vi "Get 12-bit image array.vi"(7 "Error In":errorcluster, 8 "Height":i32=2054, 9 "Width":i32=2456, 10 "Camera reference in":refnum<k24>) -> (0 "Error Out":errorcluster, 2 "Array":u16[][](array[numeric]), 3 "Camera reference out":refnum<k24>)   [LabVIEW 2017]
uses:
  C:/Program Files/National Instruments/LabVIEW 2017/instr.lib/IDS/ueye.NET/uEyeDotNet.dll
panel:
  out "Cam read time":u32
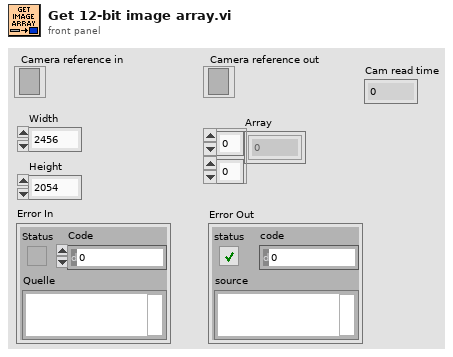
[diagram p1: front panel]
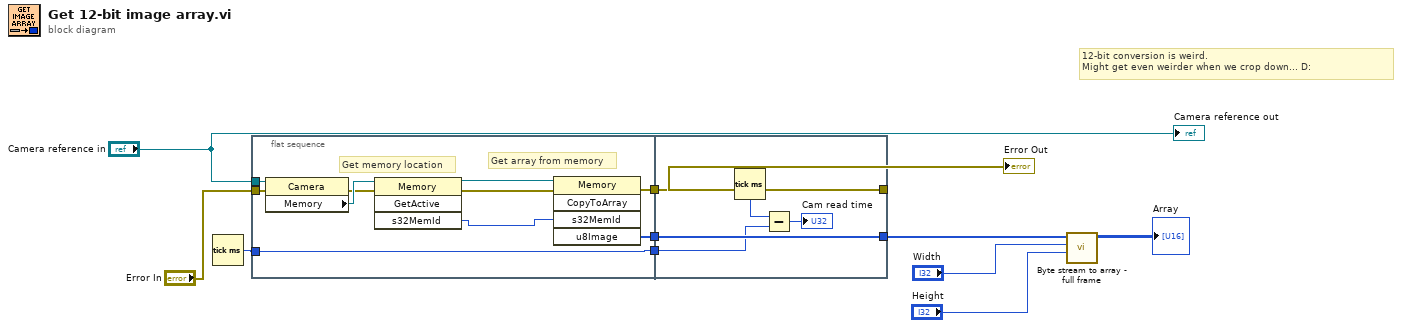
[diagram p0: block diagram]
diagram:
  # "12-bit conversion is weird.\nMight get even weirder when we crop down... D:"
  n1 = Tick Count (ms)() -> (millisecond timer value=w3:u32)
  n2 = flat-sequence {
    tunnel: "Error In" -> [w19]
    tunnel: "Camera reference in" -> [w17]
    tunnel: [w18] -> w7
    tunnel: [w14] -> w6
    tunnel: [w13] -> w4
    tunnel: w3 -> [w13]
    tunnel: [w25] -> w8
    tunnel: [w26] -> w10
    tunnel: w7 -> [w26]
    tunnel: w6 -> [w25]
    tunnel: w4 -> [w22]
    frame #0 {
      # "Get array from memory"
      # "Get memory location"
      n3 = property class="Camera"(reference=w17, error in=w19) -> (error out=w20:errorcluster, "Memory"=w21:refnum<k24>)  [unwired: 1 out]
      n4 = invoke class="Memory" method="GetActive"(reference=w21, error in=w20) -> (reference out=w16:refnum<k24>, error out=w15:errorcluster, "s32MemId"=w12:i32)  [unwired: 2 in, 1 out]
      n5 = invoke class="Memory" method="CopyToArray"(reference=w16, error in=w15, "s32MemId"=w12) -> (error out=w14:errorcluster, "u8Image"=w18:u8[])  [unwired: 2 in, 3 out]
    }
    frame #1 {
      n6 = Tick Count (ms)() -> (millisecond timer value=w23:u32)
      n7 = Subtract(x=w23, y=w22) -> (x-y=→"Cam read time":u32)
    }
  }
  n8 = call "Byte stream to array - full frame.vi"("Height"="Height", "Width"="Width", "u8Image"=w10) -> ("Array"=→"Array":u16[][])  [unwired: 8 in]
  "Error Out" <- w8
  "Camera reference out" <- "Camera reference in"
